vi "SMBUS Read Byte.vi"(7 "WithPEC":u8, 9 "SlaveAddr":i16, 10 "IICIndex":i32, 11 "DevIndex":i32) -> (2 "function return":i32, 3 "pData":u8[](array[numeric]))   [LabVIEW 2010, in "usb2iic.lvlib"]
doc: "int WINAPI SMBUS_ReadByte(int DevIndex,int IICIndex,short SlaveAddr,unsigned char *pData,unsigned char WithPEC);"
uses:
  usb2iic.lvlib
  USB2XXX.dll
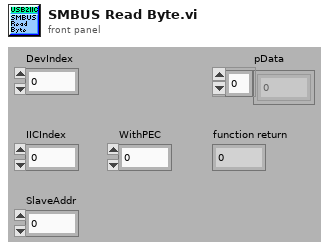
[diagram p1: front panel]
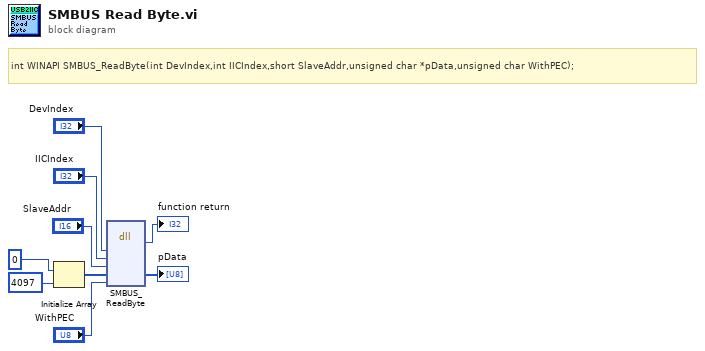
[diagram p0: block diagram]
diagram:
  # "int WINAPI SMBUS_ReadByte(int DevIndex,int IICIndex,short SlaveAddr,unsigned char *pData,unsigned char WithPEC);"
  n1 = Initialize Array(u8 0 ("element"), 4097 ("dimension size")) -> (w5:u8[])
  n2 = dll-call lib="G:/OtherWork/USB2XXX_Example/trunk/Labview/PublicFiles/usb2iic/USB2XXX.*" fn="SMBUS_ReadByte"("DevIndex"="DevIndex", "IICIndex"="IICIndex", "SlaveAddr"="SlaveAddr", "pData"=w5, "WithPEC"="WithPEC") -> (→"function return":i32, "pData"=→"pData":u8[])  [unwired: 7 in, 2 out]
